vi "String star print.vi"() -> ()   [LabVIEW 2015]
panel:
  out "concatenated string":string
  # "String value print"
  # "Pardeep Kumar"
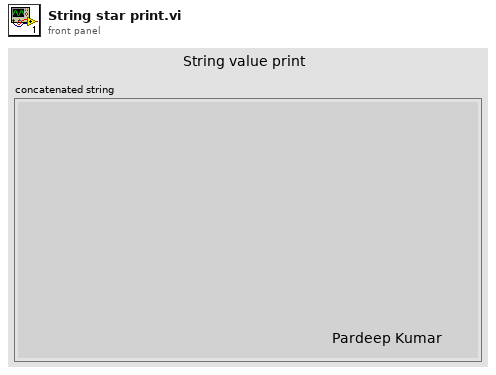
[diagram p1: front panel]
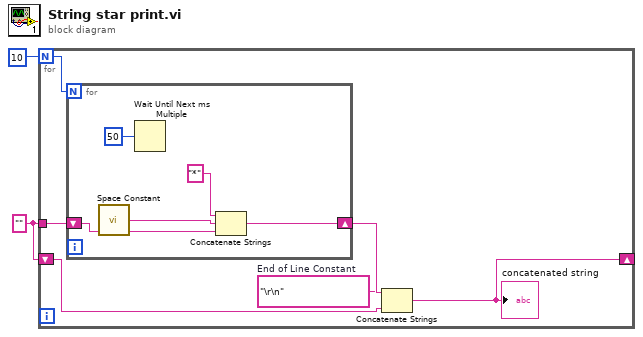
[diagram p0: block diagram]
diagram:
  w1 = ""
  n1 = for {
    N: 10 -> [w8]
    shift-right: [w6] -> _
    shift-left: w1 -> [w5]
    tunnel: w1 -> [w3]
    w4 = "\r\n"  # End of Line Constant
    n2 = for {
      N: w8 -> [_]
      shift-right: [w12] -> w7
      shift-left: w3 -> [w11]
      n3 = call <vilib>:"Space Constant.vi"() -> ("String"=w10:string)
      n4 = Wait Until Next ms Multiple(millisecond multiple=u32 50) -> ()  [unwired: 1 out]
      n5 = Concatenate Strings "Concatenate Strings"("*" ("string"), w10, w11) -> (w12:string)
    }
    n6 = Concatenate Strings "Concatenate Strings"(w7, w4, w5) -> (w6:string)
    "concatenated string" <- w6
  }
